vi "移位寄存器（累加累乘，利用反馈节点）.vi"() -> ()   [LabVIEW 2017]
panel:
  out "累乘":i32
  out "累加":i32
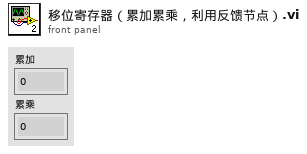
[diagram p1: front panel]
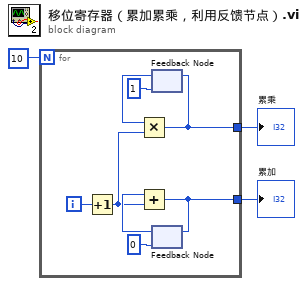
[diagram p0: block diagram]
diagram:
  n1 = for {
    N: 10 -> [_]
    tunnel: [w5] -> w1
    tunnel: [w4] -> w2
    i -> [w11]
    n2 = Increment(x=w11) -> (x+1=w8:i32)
    n3 = feedback #1(1) -> (w7:i32)
    n4 = Multiply(x=w7, y=w8) -> (x*y=w5:i32)
    n5 = feedback-in #1(w5) -> ()
    n6 = feedback #2(0) -> (w10:i32)
    n7 = Add(x=w10, y=w8) -> (x+y=w4:i32)
    n8 = feedback-in #2(w4) -> ()
  }
  "累加" <- w2
  "累乘" <- w1
